vi "写入bool_ref.vi"(8 "error in (no error)":errorcluster caption="错误输入（无错误）", 10 "布尔8 5":refnum<vi>, 11 "RandomMoveBool输入":refnum<class "RandomMoveBool.lvclass">) -> (0 "error out":errorcluster caption="错误输出", 3 "RandomMoveBool输出":refnum<class "RandomMoveBool.lvclass">)   [LabVIEW 2018, in "RandomMoveBool.lvclass"]
uses:
  RandomMoveBool.lvclass
  RandomMoveBool.lvclass/RandomMoveBool.ctl
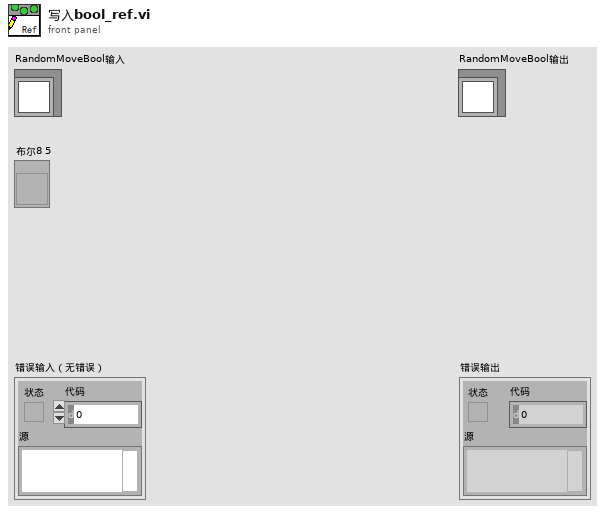
[diagram p1: front panel]
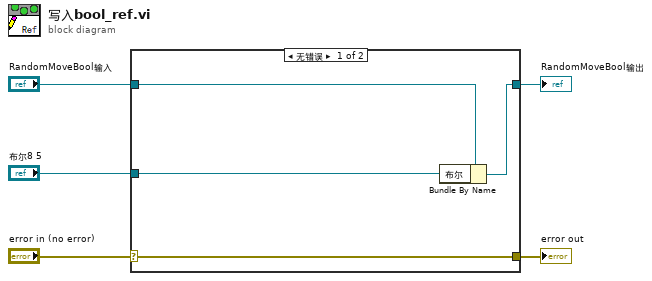
[diagram p0: block diagram]
diagram:
  n1 = case shown="无错误" "error in (no error)" {
    selector: "error in (no error)" -> [w9 w10]
    tunnel: [w9 w10] -> w4
    tunnel: [w7 w11] -> w2
    tunnel: "RandomMoveBool输入" -> [w8 w11]
    tunnel: "布尔8 5" -> [w6 _]
    frame No Error {
      n2 = Bundle By Name(cluster=w8, "布尔"=w6) -> (w7:refnum<class "RandomMoveBool.lvclass">)
    }
    frame Error {
    }
  }
  "error out" <- w4
  "RandomMoveBool输出" <- w2
